vi "Task_02.vi"() -> ()   [LabVIEW 2015]
panel:
  out "Waveform Graph":dbl[](graph)
  in  "Enum":enum16{"Экспоненциальная", "Степенная"}(ring)
  in  "Base":dbl min=0.0
  in  "Number of dots":dbl=1.0 min=1.0
  in  "Upper bound":dbl
  in  "Lower bound":dbl
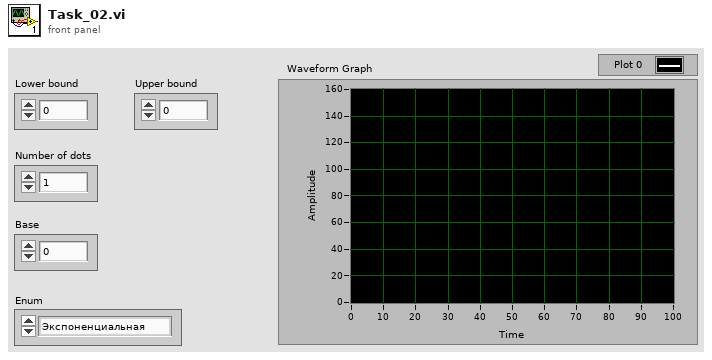
[diagram p1: front panel]
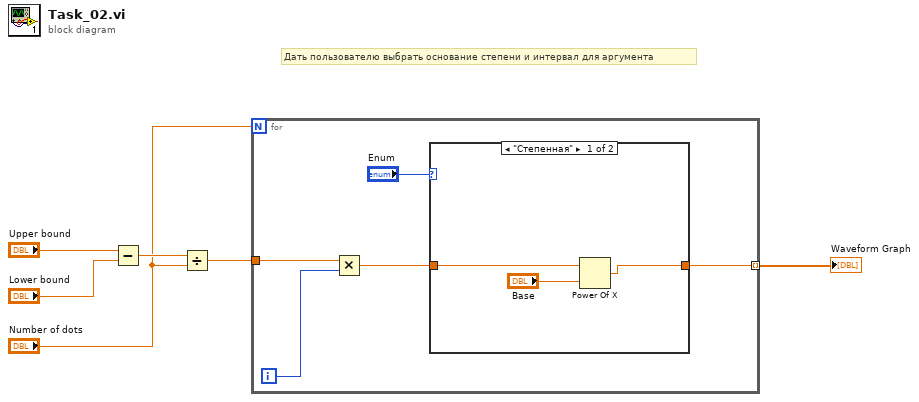
[diagram p0: block diagram]
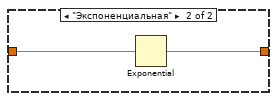
[diagram p2: hidden frame]
diagram:
  # "Дать пользователю выбрать основание степени и интервал для аргумента"
  n1 = Subtract(x="Upper bound", y="Lower bound") -> (x-y=w4:dbl)
  n2 = Divide(x=w4, y="Number of dots") -> (x/y=w3:dbl)
  n3 = for {
    N: "Number of dots" -> [_]
    tunnel: w3 -> [w10]
    tunnel: [w7] -> w1 mode=indexing
    i -> [w9]
    n4 = Multiply(x=w10, y=w9) -> (x*y=w8:dbl)
    n5 = case shown="\"Степенная\"" "Enum" {
      tunnel: w8 -> [w13 w16]
      tunnel: [w12 w15] -> w7
      frame "Степенная" {
        n6 = Power Of X(1:"Base", 2:w13) -> (0:w12:dbl)
      }
      frame "Экспоненциальная" {
        n7 = Exponential(1:w16) -> (0:w15:dbl)
      }
    }
  }
  "Waveform Graph" <- w1
